vi "Configure Settling Delay.vi"(7 "Function (0: Volts)":u16(ring) items=["Volts", "Current"], 8 "error in (no error)":errorcluster, 9 "Manual Delay (0 sec)":dbl, 10 "Auto Delay (T: Enable)":bool=TRUE, 11 "VISA resource name":refnum<visa-resource-name>) -> (0 "error out":errorcluster, 3 "VISA resource name out":refnum<visa-resource-name>)   [LabVIEW 2021, in "Keithley 2450.lvlib"]
doc: "Configures the delay between the setting of the source and the taking of the measurement."
uses:
  <instrlib>/Keithley 2450/Keithley 2450.lvlib
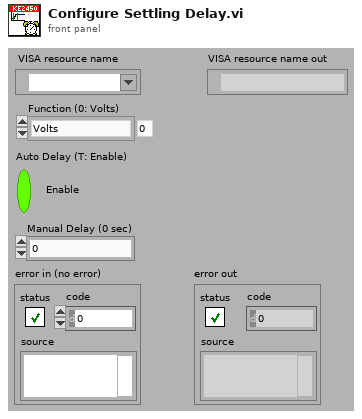
[diagram p1: front panel]
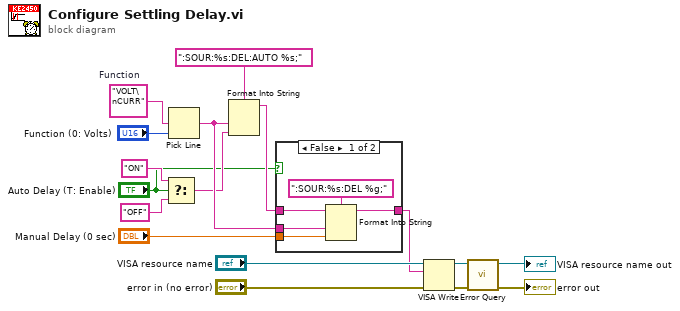
[diagram p0: block diagram]
diagram:
  w12 = "VOLT\nCURR"  # Function
  n1 = Select(t="ON", s="Auto Delay (T: Enable)", f="OFF") -> (s? t:f=w8:string)
  n2 = Pick Line(multi-line string=w12, line index="Function (0: Volts)") -> (output string=w9:string)  [unwired: 1 out]
  n3 = Format Into String(format string=":SOUR:%s:DEL:AUTO %s;", w9, w8) -> (resulting string=w2:string)  [unwired: 2 in, 1 out]
  n4 = case shown="False" "Auto Delay (T: Enable)" {
    tunnel: "Manual Delay (0 sec)" -> [w22 _]
    tunnel: w9 -> [w20 _]
    tunnel: [w19 w23] -> w3
    tunnel: w2 -> [w18 w23]
    frame False {
      n5 = Format Into String(format string=":SOUR:%s:DEL %g;", initial string=w18, w20, w22) -> (resulting string=w19:string)  [unwired: 1 in, 1 out]
    }
    frame True {
    }
  }
  n6 = VISA Write(VISA resource name="VISA resource name", write buffer=w3, error in (no error)="error in (no error)") -> (VISA resource name out=w6:refnum<visa-resource-name>, error out=w4:errorcluster)  [unwired: 1 out]
  n7 = call <instrlib>:"Error Query.vi"("error in (no error)"=w4, "VISA resource name"=w6) -> ("error out"=→"error out":errorcluster, "VISA resource name out"=→"VISA resource name out":refnum<visa-resource-name>)  [unwired: 8 out]
